vi "AI- Test GET ALL TEMP v7.vi"(0 "LA01-EN":bool, 1 "simulate":bool, 5 "LA02-EN":bool, 7 "LA03-EN":bool, 9 "LA04-EN":bool, 11 "LA05-EN":bool, 12 "Gen Cal Value":dbl) -> (2 "LOOP TIME":dbl, 3 "ID":T1, 4 "LA01 TEMP":T2, 6 "LA02 TEMP":T2, 8 "LA03 TEMP":T2, 10 "LA04 TEMP":T2, 14 "error":bool, 15 "LA05 TEMP":T2)   [LabVIEW 2013]
uses:
  program files/Global display 4.vi
panel:
  out "READ":bool
  in  "Loop mS":u32
  in  "stop":bool
  in  "COM port":refnum<visa-resource-name>="COM6"
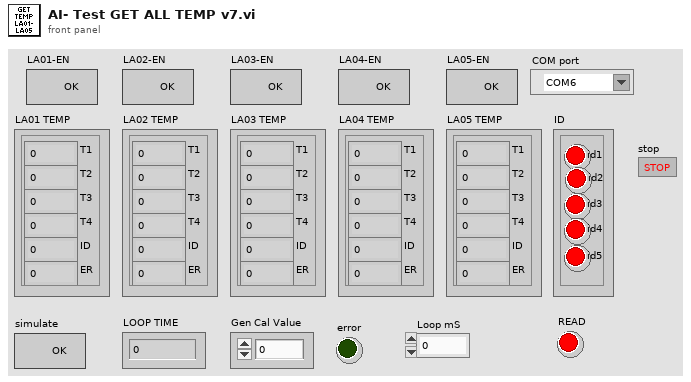
[diagram p1: front panel]
types:
  T1 = cluster{"id1":bool, "id2":bool, "id3":bool, "id4":bool, "id5":bool}
  T2 = cluster{"T1":dbl, "T2":dbl, "T3":dbl, "T4":dbl, "ID":dbl, "ER":dbl}
  T3 = cluster{"1 TL":dbl, "1 TN":dbl, "2 TL":dbl, "2 TN":dbl, "ID":dbl, "ER":dbl}
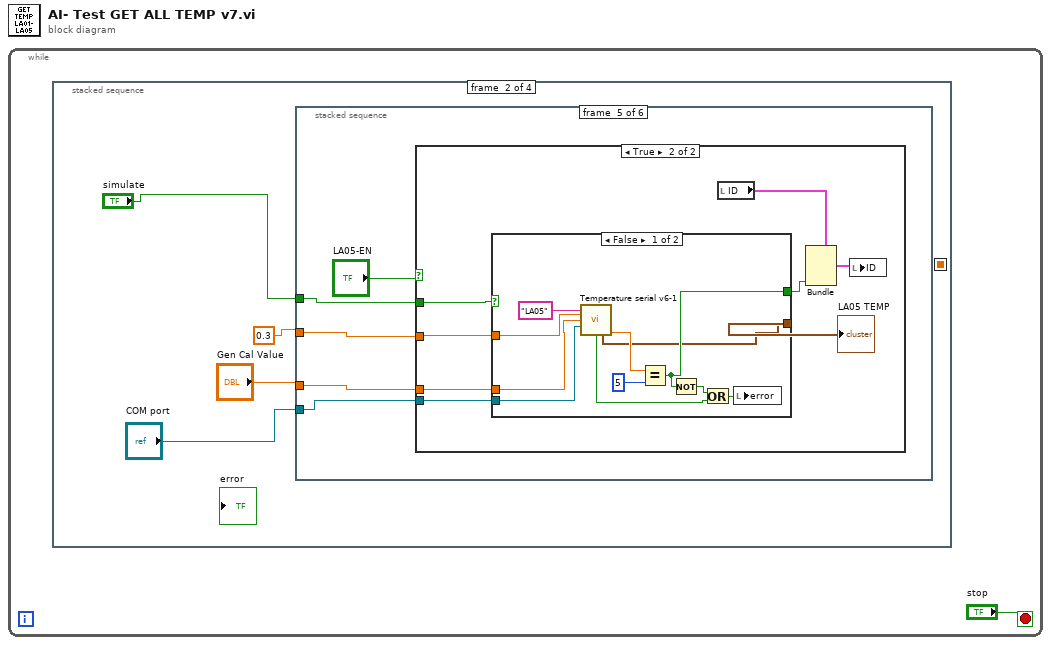
[diagram p0: block diagram]
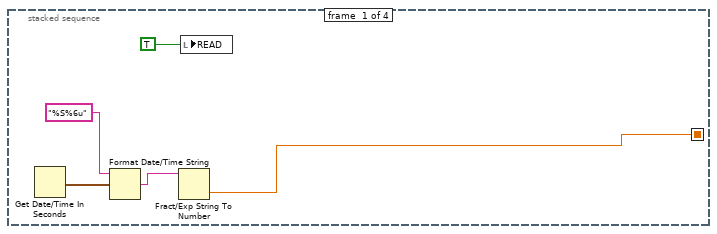
[diagram p2: hidden frame]
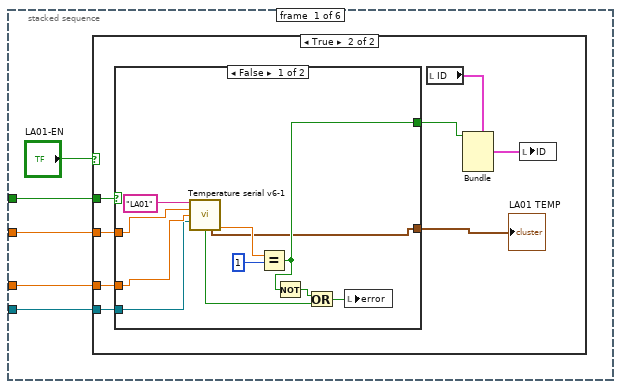
[diagram p3: hidden frame]
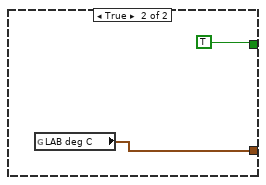
[diagram p5: hidden frame]
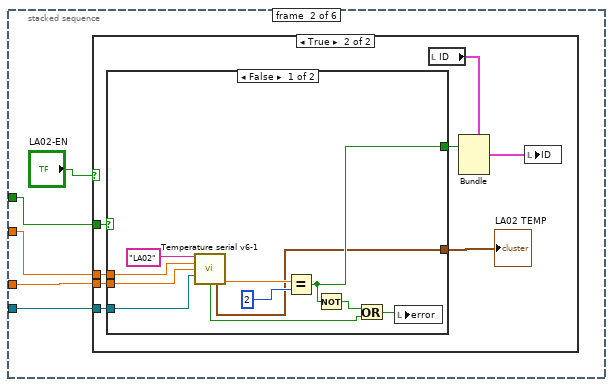
[diagram p6: hidden frame]
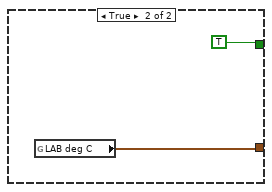
[diagram p8: hidden frame]
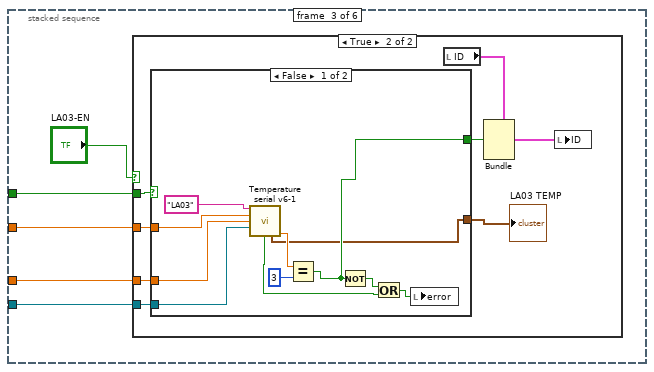
[diagram p9: hidden frame]
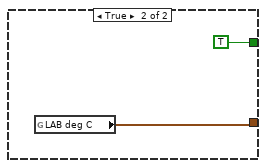
[diagram p11: hidden frame]
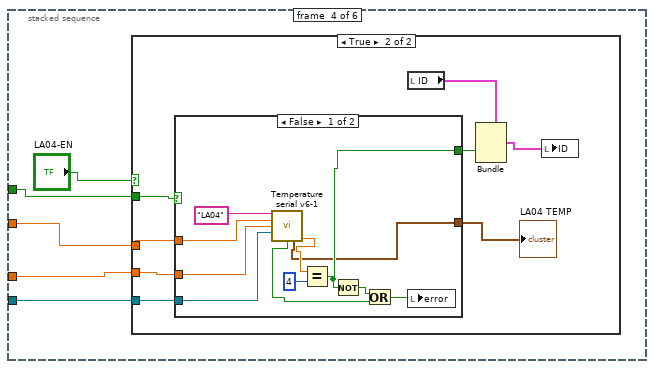
[diagram p12: hidden frame]
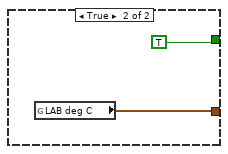
[diagram p14: hidden frame]
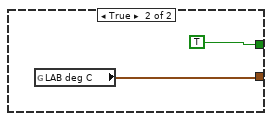
[diagram p16: hidden frame]
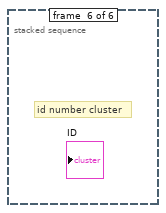
[diagram p17: hidden frame]
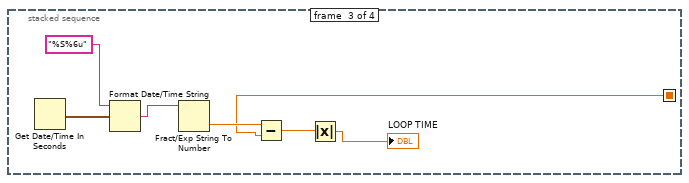
[diagram p18: hidden frame]
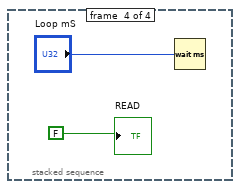
[diagram p19: hidden frame]
diagram:
  n1 = while {
    stop <- "stop" stop-if-true
    n2 = stacked-sequence {
      seq-local: [w3 _ _ _] -> [_ _ w143 _]
      frame #0 {
        n3 = Get Date/Time In Seconds() -> (seconds since 1Jan1904=w6:timestamp)
        n4 = Format Date/Time String(time format string (%c)="%S%6u", seconds (now)=w6) -> (date/time string=w4:string)  [unwired: 1 in]
        n5 = Fract/Exp String To Number(string=w4) -> (number=w3:dbl)  [unwired: 3 in, 1 out]
        n6 = local write "READ"(TRUE) -> ()
      }
      frame #1 {
        n7 = stacked-sequence {
          tunnel: 0.3 -> [w15 w41 w67 w93 w119 _]
          tunnel: "Gen Cal Value" -> [w14 w40 w66 w92 w118 _]
          tunnel: "simulate" -> [w12 w38 w64 w90 w116 _]
          tunnel: "COM port" -> [w11 w37 w63 w89 w115 _]
          frame #0 {
            n8 = case shown="True" "LA01-EN" {
              tunnel: w15 -> [_ w23]
              tunnel: w14 -> [_ w22]
              tunnel: w12 -> [_ w20]
              tunnel: w11 -> [_ w16]
              frame False {
              }
              frame True {
                n9 = case shown="False" w20 {
                  tunnel: w23 -> [w29 _]
                  tunnel: w22 -> [w28 _]
                  tunnel: [w25 w36] -> w21
                  tunnel: [w31 TRUE] -> w19
                  tunnel: w16 -> [w27 _]
                  frame False {
                    n10 = call "Temperature serial v6-1.vi"("Command String"="LA01", "Time Out (S)"=w29, "CALIB"=w28, "COM port"=w27) -> ("error"=w24:bool, "output cluster"=w25:cluster{dbl, dbl, dbl, dbl, i32, "error #":dbl}, "Unit ID"=w26:dbl)  [unwired: 5 in, 4 out]
                    n11 = Equal?(x=w26, y=1) -> (x = y?=w31:bool)
                    n12 = Not(x=w31) -> (.not. x?=w32:bool)
                    n13 = Or(x=w32, y=w24) -> (x .or. y?=w33:bool)
                    n14 = local write "error"(w33) -> ()
                  }
                  frame True {
                    n15 = global read "Global display 4.vi" "LAB deg C"() -> (w36:T3)
                  }
                }
                "LA01 TEMP" <- w21
                n16 = local read "ID"() -> (w18:T1)
                n17 = Bundle(cluster=w18, "id1"=w19) -> (w17:T1)  [unwired: 4 in]
                n18 = local write "ID"(w17) -> ()
              }
            }
          }
          frame #1 {
            n19 = case shown="True" "LA02-EN" {
              tunnel: w41 -> [_ w49]
              tunnel: w40 -> [_ w48]
              tunnel: w38 -> [_ w46]
              tunnel: w37 -> [_ w42]
              frame False {
              }
              frame True {
                n20 = case shown="False" w46 {
                  tunnel: w49 -> [w55 _]
                  tunnel: w48 -> [w54 _]
                  tunnel: [w51 w62] -> w47
                  tunnel: [w57 TRUE] -> w45
                  tunnel: w42 -> [w53 _]
                  frame False {
                    n21 = call "Temperature serial v6-1.vi"("Command String"="LA02", "Time Out (S)"=w55, "CALIB"=w54, "COM port"=w53) -> ("error"=w50:bool, "output cluster"=w51:cluster{dbl, dbl, dbl, dbl, i32, "error #":dbl}, "Unit ID"=w52:dbl)  [unwired: 5 in, 4 out]
                    n22 = Equal?(x=w52, y=2) -> (x = y?=w57:bool)
                    n23 = Not(x=w57) -> (.not. x?=w58:bool)
                    n24 = Or(x=w58, y=w50) -> (x .or. y?=w60:bool)
                    n25 = local write "error"(w60) -> ()
                  }
                  frame True {
                    n26 = global read "Global display 4.vi" "LAB deg C"() -> (w62:T3)
                  }
                }
                "LA02 TEMP" <- w47
                n27 = local read "ID"() -> (w44:T1)
                n28 = Bundle(cluster=w44, "id2"=w45) -> (w43:T1)  [unwired: 4 in]
                n29 = local write "ID"(w43) -> ()
              }
            }
          }
          frame #2 {
            n30 = case shown="True" "LA03-EN" {
              tunnel: w67 -> [_ w75]
              tunnel: w66 -> [_ w74]
              tunnel: w64 -> [_ w72]
              tunnel: w63 -> [_ w68]
              frame False {
              }
              frame True {
                n31 = case shown="False" w72 {
                  tunnel: w75 -> [w81 _]
                  tunnel: w74 -> [w80 _]
                  tunnel: [w77 w88] -> w73
                  tunnel: [w83 TRUE] -> w71
                  tunnel: w68 -> [w79 _]
                  frame False {
                    n32 = call "Temperature serial v6-1.vi"("Command String"="LA03", "Time Out (S)"=w81, "CALIB"=w80, "COM port"=w79) -> ("error"=w76:bool, "output cluster"=w77:cluster{dbl, dbl, dbl, dbl, i32, "error #":dbl}, "Unit ID"=w78:dbl)  [unwired: 5 in, 4 out]
                    n33 = Equal?(x=w78, y=3) -> (x = y?=w83:bool)
                    n34 = Not(x=w83) -> (.not. x?=w84:bool)
                    n35 = Or(x=w84, y=w76) -> (x .or. y?=w86:bool)
                    n36 = local write "error"(w86) -> ()
                  }
                  frame True {
                    n37 = global read "Global display 4.vi" "LAB deg C"() -> (w88:T3)
                  }
                }
                "LA03 TEMP" <- w73
                n38 = local read "ID"() -> (w70:T1)
                n39 = Bundle(cluster=w70, "id3"=w71) -> (w69:T1)  [unwired: 4 in]
                n40 = local write "ID"(w69) -> ()
              }
            }
          }
          frame #3 {
            n41 = case shown="True" "LA04-EN" {
              tunnel: w93 -> [_ w101]
              tunnel: w92 -> [_ w100]
              tunnel: w90 -> [_ w98]
              tunnel: w89 -> [_ w94]
              frame False {
              }
              frame True {
                n42 = case shown="False" w98 {
                  tunnel: w101 -> [w107 _]
                  tunnel: w100 -> [w106 _]
                  tunnel: [w103 w114] -> w99
                  tunnel: [w109 TRUE] -> w97
                  tunnel: w94 -> [w105 _]
                  frame False {
                    n43 = call "Temperature serial v6-1.vi"("Command String"="LA04", "Time Out (S)"=w107, "CALIB"=w106, "COM port"=w105) -> ("error"=w102:bool, "output cluster"=w103:cluster{dbl, dbl, dbl, dbl, i32, "error #":dbl}, "Unit ID"=w104:dbl)  [unwired: 5 in, 4 out]
                    n44 = Equal?(x=w104, y=4) -> (x = y?=w109:bool)
                    n45 = Not(x=w109) -> (.not. x?=w110:bool)
                    n46 = Or(x=w110, y=w102) -> (x .or. y?=w112:bool)
                    n47 = local write "error"(w112) -> ()
                  }
                  frame True {
                    n48 = global read "Global display 4.vi" "LAB deg C"() -> (w114:T3)
                  }
                }
                "LA04 TEMP" <- w99
                n49 = local read "ID"() -> (w96:T1)
                n50 = Bundle(cluster=w96, "id4"=w97) -> (w95:T1)  [unwired: 4 in]
                n51 = local write "ID"(w95) -> ()
              }
            }
          }
          frame #4 {
            n52 = case shown="True" "LA05-EN" {
              tunnel: w119 -> [_ w127]
              tunnel: w118 -> [_ w126]
              tunnel: w116 -> [_ w124]
              tunnel: w115 -> [_ w120]
              frame False {
              }
              frame True {
                n53 = case shown="False" w124 {
                  tunnel: w127 -> [w133 _]
                  tunnel: w126 -> [w132 _]
                  tunnel: [w129 w140] -> w125
                  tunnel: [w135 TRUE] -> w123
                  tunnel: w120 -> [w131 _]
                  frame False {
                    n54 = call "Temperature serial v6-1.vi"("Command String"="LA05", "Time Out (S)"=w133, "CALIB"=w132, "COM port"=w131) -> ("error"=w128:bool, "output cluster"=w129:cluster{dbl, dbl, dbl, dbl, i32, "error #":dbl}, "Unit ID"=w130:dbl)  [unwired: 5 in, 4 out]
                    n55 = Equal?(x=w130, y=5) -> (x = y?=w135:bool)
                    n56 = Not(x=w135) -> (.not. x?=w136:bool)
                    n57 = Or(x=w136, y=w128) -> (x .or. y?=w138:bool)
                    n58 = local write "error"(w138) -> ()
                  }
                  frame True {
                    n59 = global read "Global display 4.vi" "LAB deg C"() -> (w140:T3)
                  }
                }
                "LA05 TEMP" <- w125
                n60 = local read "ID"() -> (w122:T1)
                n61 = Bundle(cluster=w122, "id5"=w123) -> (w121:T1)  [unwired: 4 in]
                n62 = local write "ID"(w121) -> ()
              }
            }
          }
          frame #5 {
            # "id number cluster"
          }
        }
      }
      frame #2 {
        n63 = Get Date/Time In Seconds() -> (seconds since 1Jan1904=w147:timestamp)
        n64 = Format Date/Time String(time format string (%c)="%S%6u", seconds (now)=w147) -> (date/time string=w145:string)  [unwired: 1 in]
        n65 = Fract/Exp String To Number(string=w145) -> (number=w144:dbl)  [unwired: 3 in, 1 out]
        n66 = Subtract(x=w144, y=w143) -> (x-y=w142:dbl)
        n67 = Absolute Value(x=w142) -> (abs(x)=→"LOOP TIME":dbl)
      }
      frame #3 {
        n68 = Wait (ms)(milliseconds to wait="Loop mS") -> ()  [unwired: 1 out]
        "READ" <- FALSE
      }
    }
  }
